vi "Module仪器串口通讯.vi"(3 "输入指令":string, 4 "baud rate":u32=300, 5 "VISA resource name":refnum<visa-resource-name>="COM3") -> (0 "错误输出":errorcluster, 1 "read buffer":string, 2 "子字符串;substring":string)   [LabVIEW 2016]
uses:
  <vilib>/Instr/_visa.llb/VISA Configure Serial Port (Instr).vi
panel:
  out "输入的字符串":string
  out "返回数 2":u32
  out "返回数":u32
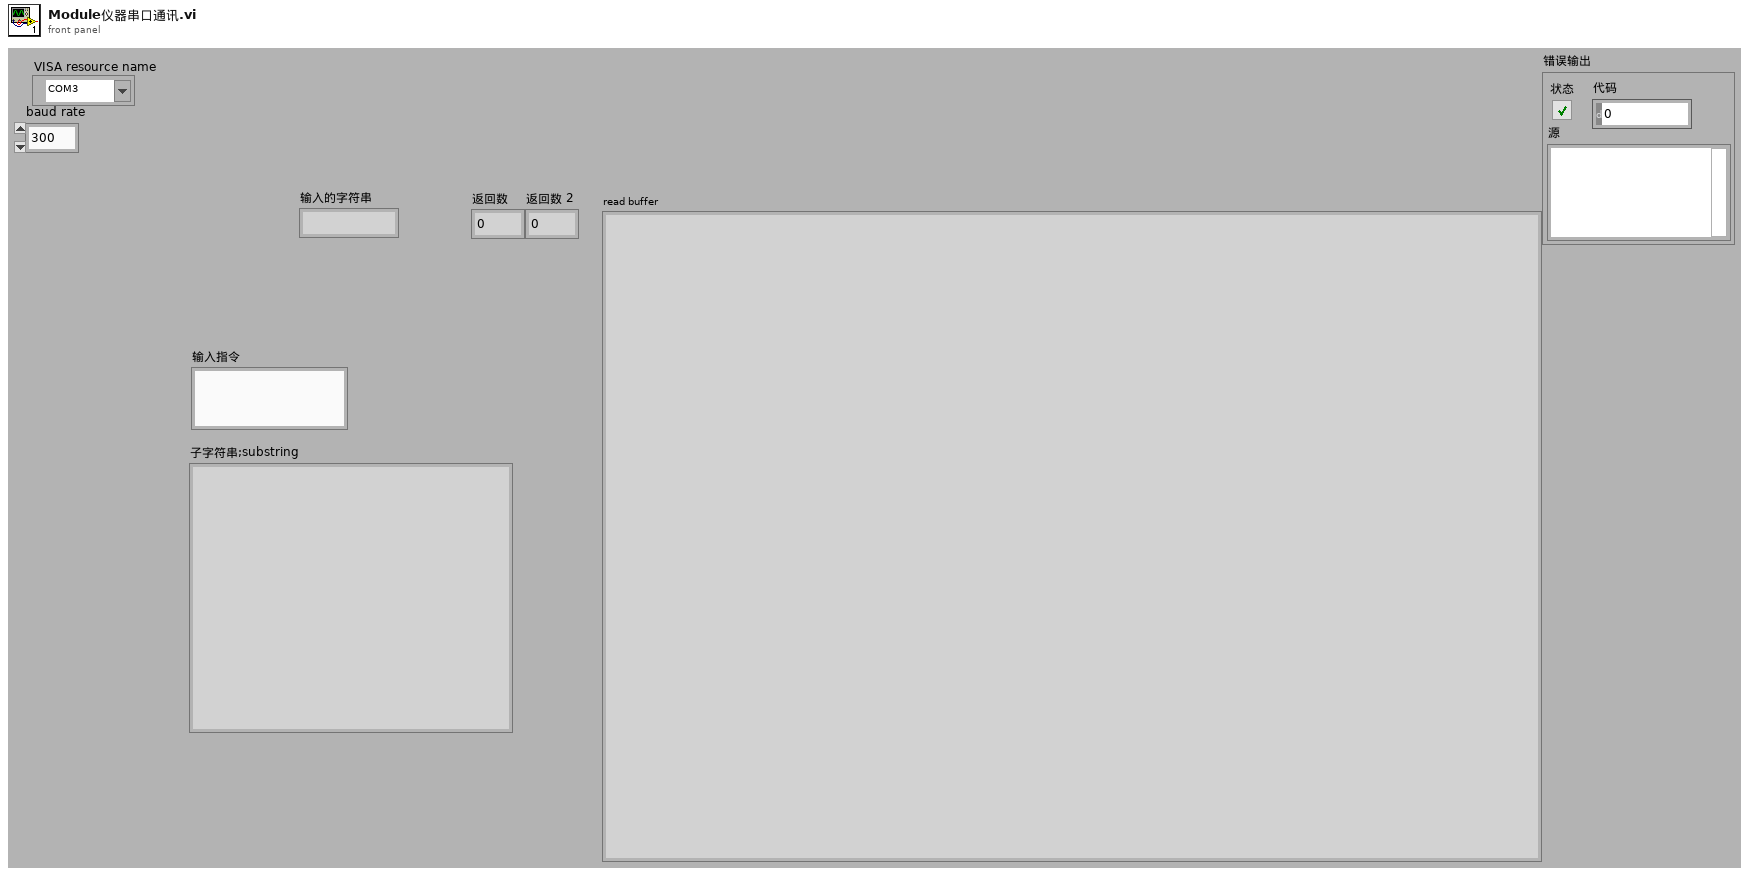
[diagram p1: front panel]
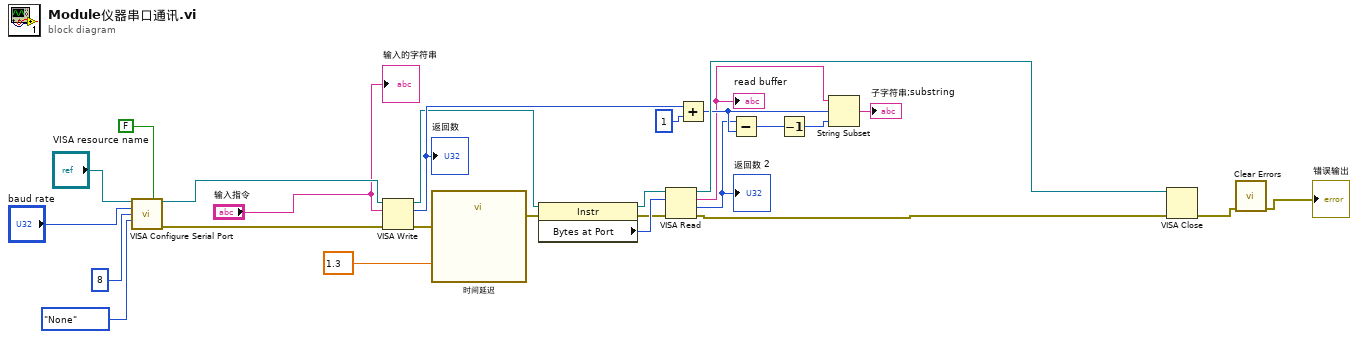
[diagram p0: block diagram]
diagram:
  n1 = call-poly "VISA Configure Serial Port"("VISA resource name"="VISA resource name", "Enable Termination\nChar (T)"=FALSE ("Enable Termination\nChar (T)"), "baud rate (9600)"="baud rate", "data bits (8)"=u16 8, "parity (0:none)"=enum16{"None", "Odd", "Even", "Mark", "Space"}."None") -> ("VISA resource name out"=w24:refnum<visa-resource-name>, "error out"=w23:errorcluster)  [unwired: 9 in]
  n2 = VISA Write(VISA resource name=w24, write buffer="输入指令", error in (no error)=w23) -> (VISA resource name out=w6:refnum<visa-resource-name>, return count=w11:u32, error out=w19:errorcluster)
  "返回数" <- w11
  n3 = call "时间延迟"("error in (no error)"=w19, "Delay Time (s)"=1.3) -> ("error out"=w18:errorcluster)  [unwired: 9 in]
  n4 = property class="Instr"(reference=w6, error in=w18) -> (reference out=w15:refnum<visa-resource-name>, error out=w16:errorcluster, "Bytes at Port"=w17:u32)
  n5 = VISA Read(VISA resource name=w15, byte count=w17, error in (no error)=w16) -> (VISA resource name out=w21:refnum<visa-resource-name>, read buffer=w10:string, return count=w9:u32, error out=w22:errorcluster)
  "read buffer" <- w10
  "返回数 2" <- w9
  n6 = Add(x=w11, y=1 ("偏移量(0)")) -> (x+y=w13:u32)
  n7 = Subtract(x=w9, y=w13) -> (x-y=w7:u32)
  n8 = Decrement(x=w7) -> (x-1=w8:u32)
  n9 = String Subset(string=w10, offset (0)=w13, length (rest)=w8) -> (substring=→"子字符串;substring":string)
  n10 = VISA Close(VISA resource name=w21, error in (no error)=w22) -> (error out=w3:errorcluster)
  n11 = call <vilib>:"Clear Errors.vi"("error in (no error)"=w3) -> ("error out"=→"错误输出":errorcluster)  [unwired: 5 in, 1 out]
  "输入的字符串" <- "输入指令"
